vi "MetaInfo.vi"(8 "error in (no error)":errorcluster, 10 "meta info":refnum<k24>, 11 "VGS_MetaInfo in":refnum<class "VGS_MetaInfo.lvclass">) -> (0 "error out":errorcluster, 3 "VGS_MetaInfo out":refnum<class "VGS_MetaInfo.lvclass">)   [LabVIEW 2022 SP3, in "LV_VGS.lvlib" / "VGS_MetaInfo.lvclass"]
uses:
  VGS_MetaInfo.lvclass
  C:/Users/Andrey/Documents/GitHub/LV_VGS/vgs_project.dll
  vgs_project.dll
  VGS_MetaInfo.lvclass/VGS_MetaInfo.ctl
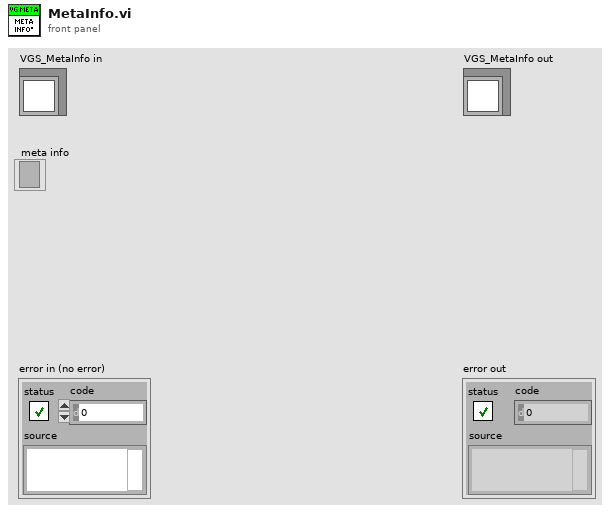
[diagram p1: front panel]
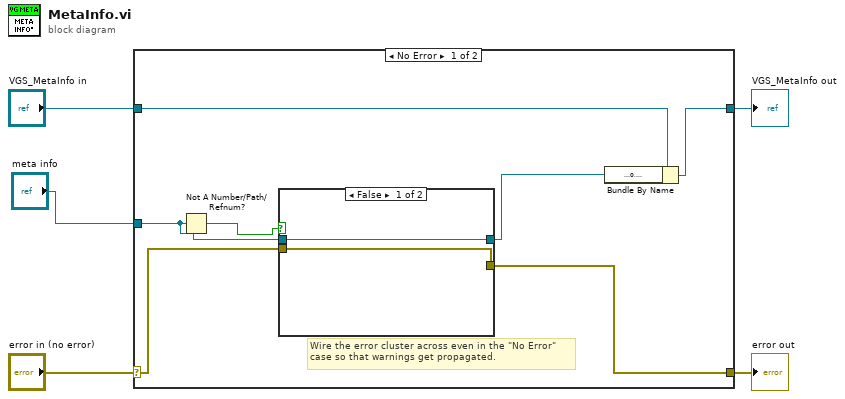
[diagram p0: block diagram]
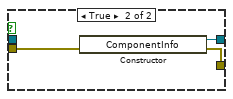
[diagram p2: hidden frame]
diagram:
  n1 = case shown="No Error" "error in (no error)" {
    selector: "error in (no error)" -> [w7 w19]
    tunnel: [w6 w19] -> w4
    tunnel: [w11 w18] -> w2
    tunnel: "VGS_MetaInfo in" -> [w12 w18]
    tunnel: "meta info" -> [w9 _]
    frame No Error {
      # "Wire the error cluster across even in the \"No Error\"\ncase so that warnings get propagated."
      n2 = Not A Number/Path/Refnum?(number/path/refnum=w9) -> (NaN/Path/Refnum?=w10:bool)
      n3 = case shown="False" w10 {
        tunnel: [w14 w17] -> w8
        tunnel: w7 -> [w13 w16]
        tunnel: [w13 w15] -> w6
        tunnel: w9 -> [w14 _]
        frame False {
        }
        frame True {
          n4 = constructor class="ComponentInfo"(error in=w16) -> (reference out=w17:refnum<k24>, error out=w15:errorcluster)  [unwired: 2 in, 1 out]
        }
      }
      n5 = Bundle By Name(cluster=w12, "meta info"=w8) -> (w11:refnum<class "VGS_MetaInfo.lvclass">)
    }
    frame Error {
    }
  }
  "error out" <- w4
  "VGS_MetaInfo out" <- w2
